vi "Test__Zoom Corection.vi"(0 "Reference Image IN":T2, 1 "Interpolation Type":u32(ring) items=["Zero Order", "Bi-Linear", "Quadratic", "Cubic Spline"], 5 "Modified Image IN":T2, 7 "Flipped?":bool, 9 "X-Stretch":dbl, 11 "Y-Stretch":dbl, 12 "X Indices IN":i16[](array[numeric]), 13 "Y Indices IN":i16[](array[numeric])) -> (4 "Modified Image OUT":T2, 6 "X Indices OUT":i16[](array[numeric]), 8 "Y Indices OUT":i16[](array[numeric]), 10 "X_Pixels Dropped (if ZOOM <1)":T1)   [LabVIEW 2012]
uses:
  <vilib>/vision/Image Controls.llb/IMAQ Image.ctl
  <vilib>/vision/NI_Vision_Development_Module.lvlib
panel:
  out "Y Pixels after correction and trimming":i32
  out "X Pixels after correction and trimming":i32
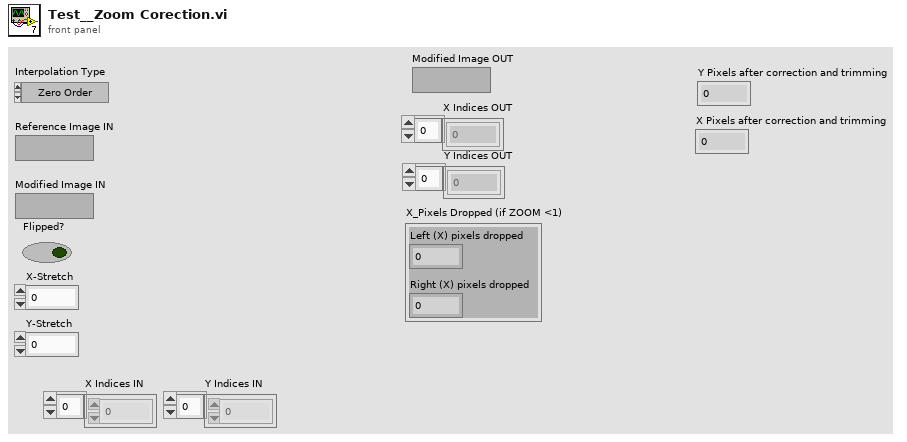
[diagram p1: front panel]
types:
  T1 = cluster{"Left (X) pixels dropped":i32, "Right (X) pixels dropped":i32}
  T2 = typedef "IMAQ Image.ctl" = refnum<image>
  T3 = typedef "Image Type" = u32
  T4 = cluster{"Left Pixels dropped":i32, "Right Pixels dropped":i32}
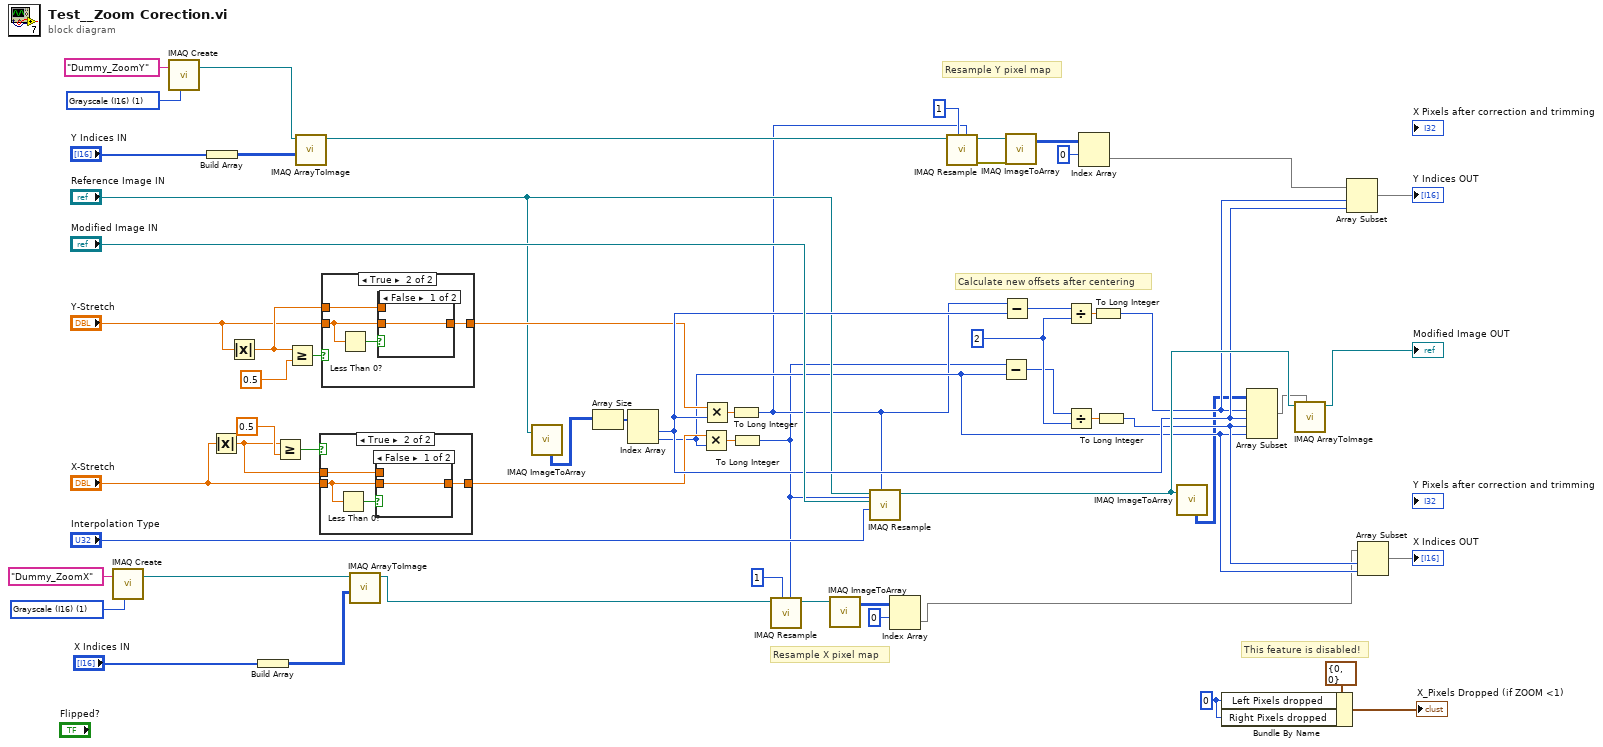
[diagram p0: block diagram]
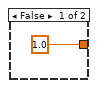
[diagram p2: hidden frame]
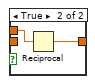
[diagram p3: hidden frame]
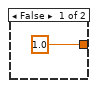
[diagram p4: hidden frame]
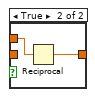
[diagram p5: hidden frame]
diagram:
  w8 = 0 ("Left Pixels dropped")
  w28 = T3 1 items=["Grayscale (U8)", "Grayscale (I16)", "Grayscale (SGL)", "Complex (CSG)", "RGB (U32)", "HSL (U32)", "RGB (U64)", "Grayscale (U16)"] ("Image Type")
  w30 = T3 1 items=["Grayscale (U8)", "Grayscale (I16)", "Grayscale (SGL)", "Complex (CSG)", "RGB (U32)", "HSL (U32)", "RGB (U64)", "Grayscale (U16)"] ("Image Type")
  w58 = 2 ("y")
  # "Calculate new offsets after centering"
  # "This feature is disabled!"
  # "Resample X pixel map"
  # "Resample Y pixel map"
  n1 = call "IMAQ Create"("Image Name"="Dummy_ZoomX", "Image Type"=w28) -> ("New Image"=w26:T2)  [unwired: 3 in, 1 out]
  n2 = call "IMAQ Create"("Image Name"="Dummy_ZoomY", "Image Type"=w30) -> ("New Image"=w29:T2)  [unwired: 3 in, 1 out]
  n3 = Build Array("Y Indices IN") -> (w19:i16[][])
  n4 = Absolute Value(x="X-Stretch") -> (abs(x)=w48:dbl)
  n5 = Absolute Value(x="Y-Stretch") -> (abs(x)=w49:dbl)
  n6 = Build Array("X Indices IN") -> (w25:i16[][])
  n7 = Greater Or Equal?(x=w48, y=0.5) -> (x >= y?=w51:bool)
  n8 = Greater Or Equal?(x=w49, y=0.5) -> (x >= y?=w52:bool)
  n9 = call "IMAQ ArrayToImage"("Image Pixels (I16)"=w19, "Image"=w29) -> ("Image Out"=w22:T2)  [unwired: 8 in, 1 out]
  n10 = case shown="True" w51 {
    tunnel: "X-Stretch" -> [_ w63]
    tunnel: [sgl 1.0 ("y") w65] -> w35
    tunnel: w48 -> [_ w62]
    frame False {
    }
    frame True {
      n11 = Less Than 0?(x=w63) -> (x < 0?=w64:bool)
      n12 = case shown="False" w64 {
        tunnel: [w66 w68] -> w65
        tunnel: w63 -> [w66 _]
        tunnel: w62 -> [_ w67]
        frame False {
        }
        frame True {
          n13 = Reciprocal(x=w67) -> (1/x=w68:dbl)
        }
      }
    }
  }
  n14 = case shown="True" w52 {
    tunnel: "Y-Stretch" -> [_ w71]
    tunnel: [sgl 1.0 ("y") w73] -> w34
    tunnel: w49 -> [_ w70]
    frame False {
    }
    frame True {
      n15 = Less Than 0?(x=w71) -> (x < 0?=w72:bool)
      n16 = case shown="False" w72 {
        tunnel: [w74 w76] -> w73
        tunnel: w71 -> [w74 _]
        tunnel: w70 -> [_ w75]
        frame False {
        }
        frame True {
          n17 = Reciprocal(x=w75) -> (1/x=w76:dbl)
        }
      }
    }
  }
  n18 = call "IMAQ ArrayToImage"("Image Pixels (I16)"=w25, "Image"=w26) -> ("Image Out"=w12:T2)  [unwired: 8 in, 1 out]
  n19 = call "IMAQ ImageToArray"("Image"="Reference Image IN") -> ("Image Pixels (U16)"=w1:u16[][])  [unwired: 3 in, 4 out]
  n20 = Array Size(array=w1) -> (size(s)=w54:i32[])
  n21 = Index Array(array=w54) -> (element #1=w42:i32, element #2=w23:i32)  [unwired: 2 in]
  n22 = Multiply(x=w35, y=w23) -> (x*y=w55:dbl)
  n23 = Multiply(x=w34, y=w42) -> (x*y=w56:dbl)
  n24 = To Long Integer(number=w56) -> (32bit integer=w17:i32)
  n25 = To Long Integer(number=w55) -> (32bit integer=w11:i32)
  n26 = call "IMAQ Resample"("X Resolution"=w11, "Y Resolution"=1 ("X Resolution"), "Image Src"=w12) -> ("Image Dst Out"=w13:T2)  [unwired: 7 in, 1 out]
  n27 = call "IMAQ ImageToArray"("Image"=w13) -> ("Image Pixels (I16)"=w15:i16[][])  [unwired: 3 in, 4 out]
  n28 = call "IMAQ Resample"("X Resolution"=w11, "Y Resolution"=w17, "Interpolation Type"="Interpolation Type", "Image Dst"="Modified Image IN", "Image Src"="Reference Image IN") -> ("Image Dst Out"=w46:T2)  [unwired: 5 in, 1 out]
  n29 = Index Array(array=w15, index (row)=0) -> (element=w5:i16[])  [unwired: 1 in]
  n30 = call "IMAQ Resample"("X Resolution"=w17, "Y Resolution"=1 ("X Resolution"), "Image Src"=w22) -> ("error out"=w21:errorcluster, "Image Dst Out"=w20:T2)  [unwired: 7 in]
  n31 = Subtract(x=w11, y=w23) -> (x-y=w36:i32)
  n32 = Subtract(x=w17, y=w42) -> (x-y=w37:i32)
  n33 = call "IMAQ ImageToArray"("error in (no error)"=w21, "Image"=w20) -> ("Image Pixels (I16)"=w16:i16[][])  [unwired: 2 in, 4 out]
  n34 = Divide(x=w37, y=w58) -> (x/y=w43:dbl)
  n35 = Divide(x=w36, y=w58) -> (x/y=w59:dbl)
  n36 = Index Array(array=w16, index (row)=0) -> (element=w4:i16[])  [unwired: 1 in]
  n37 = To Long Integer(number=w43) -> (32bit integer=w32:i32)
  n38 = To Long Integer(number=w59) -> (32bit integer=w33:i32)
  n39 = call "IMAQ ImageToArray"("Image"=w46) -> ("Image Pixels (U16)"=w3:u16[][])  [unwired: 3 in, 4 out]
  n40 = Bundle By Name(cluster=T4 {"Left Pixels dropped"=0, "Right Pixels dropped"=0} ("X and Y pixel offsets"), "Left Pixels dropped"=w8, "Right Pixels dropped"=w8) -> (→"X_Pixels Dropped (if ZOOM <1)":T4)
  n41 = Array Subset(array=w3, index (row)=w32, length (row)=w42, index (col)=w33, length (col)=w23) -> (w2:u16[][])
  n42 = call "IMAQ ArrayToImage"("Image Pixels (U16)"=w2, "Image"=w46) -> ("Image Out"=→"Modified Image OUT":T2)  [unwired: 8 in, 1 out]
  n43 = Array Subset(array=w4, index=w32, length=w42) -> (→"Y Indices OUT":i16[])
  n44 = Array Subset(array=w5, index=w33, length=w23) -> (→"X Indices OUT":i16[])
